vi "Panel Picture FGV.vi"(0 "Panel Picture Command":T1=enum."Set Update Picture", 7 "Panel Picture path in":path) -> (4 "Action":T2=enum."Update Picture", 8 "Panel Picture path out":path)   [LabVIEW 2013, in "Manipulate IPF.lvlib"]
uses:
  Manipulate IPF.lvlib
  type_def/Picture FGV actions.ctl
  type_def/Picture FGV commands.ctl
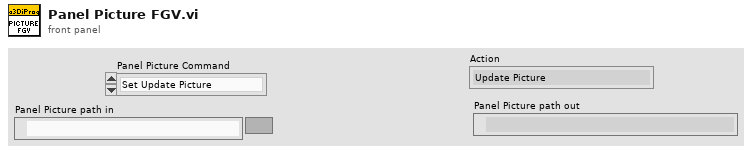
[diagram p1: front panel]
types:
  T1 = typedef "Manipulate IPF.lvlib/Picture FGV commands.ctl" = enum16{"No Action", "Set Update Picture", "Set Delete Picture", "Get Picture action"}
  T2 = typedef "Manipulate IPF.lvlib/Picture FGV actions.ctl" = enum16{"No Action", "Update Picture", "Delete Picture"}
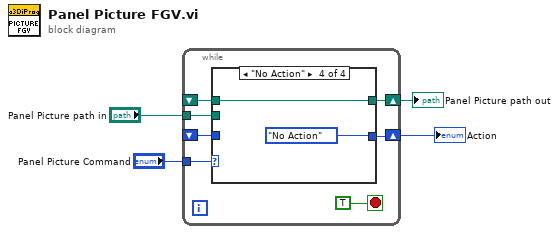
[diagram p0: block diagram]
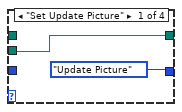
[diagram p2: hidden frame]
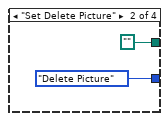
[diagram p3: hidden frame]
diagram:
  n1 = while {
    shift-right: [w11] -> w3
    shift-left: _ -> [w8]
    tunnel: "Panel Picture Command" -> [w9]
    shift-right: [w6] -> w4
    shift-left: _ -> [w7]
    tunnel: "Panel Picture path in" -> [w5]
    stop <- TRUE stop-if-true
    n2 = case shown="\"No Action\"" w9 {
      tunnel: [Picture_FGV_actions."Update Picture" Picture_FGV_actions."Delete Picture" w17 Picture_FGV_actions."No Action"] -> w11
      tunnel: w8 -> [_ _ w17 _]
      tunnel: w7 -> [_ _ w16 w18]
      tunnel: [w12 path "" w16 w18] -> w6
      tunnel: w5 -> [w12 _ _ _]
      frame "Set Update Picture" {
      }
      frame "Set Delete Picture" {
      }
      frame "Get Picture action" {
      }
      frame "No Action" {
      }
    }
  }
  "Panel Picture path out" <- w4
  "Action" <- w3
